vi "Encode Error Listbox.vi"(8 "error in (no error)":errorcluster, 11 "Data":variant) -> (0 "error out":errorcluster, 3 "Encoded Msg":string[](array[string]))   [LabVIEW 2026, in "TALOS.lvlib" / "Guardian.lvlib" / "Guardian.lvclass"]
uses:
  Guardian.lvclass
  Internal uServices/System uServices/Common GUI v3/Common GUI v3/Error Listbox Msg.ctl
  Internal uServices/System uServices/Common GUI v3/Common GUI v3/Error Listbox Msg Action.ctl
  Internal uServices/System uServices/Error Manager/Error Info.ctl
  Internal uServices/System uServices/Common GUI v3/Common GUI v3/Common GUI v3.lvclass
  Internal uServices/System uServices/Error Manager/Error Manager.lvclass
  TALOS.lvlib
  <vilib>/MultiError/TokenizeJSON/Multi Error Cluster.lvlib
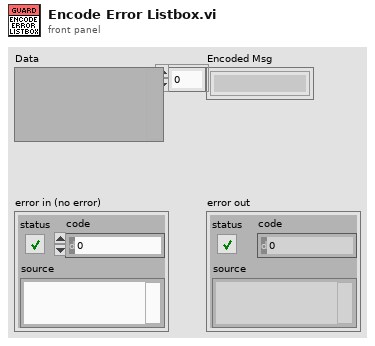
[diagram p1: front panel]
types:
  T1 = typedef "TALOS.lvlib/Common GUI v3.lvlib/Common GUI v3.lvclass/Error Listbox Msg.ctl" = cluster{"Action":T2, "Error Info":T3}
  T2 = typedef "TALOS.lvlib/Common GUI v3.lvlib/Common GUI v3.lvclass/Error Listbox Msg Action.ctl" = enum16{"Add", "Remove", "Clear"}
  T3 = typedef "TALOS.lvlib/Error Manager.lvlib/Error Manager.lvclass/Error Info.ctl" = cluster{"error out":errorcluster, "Time Stamp":timestamp, "Machine Name":string, "GUID":string}
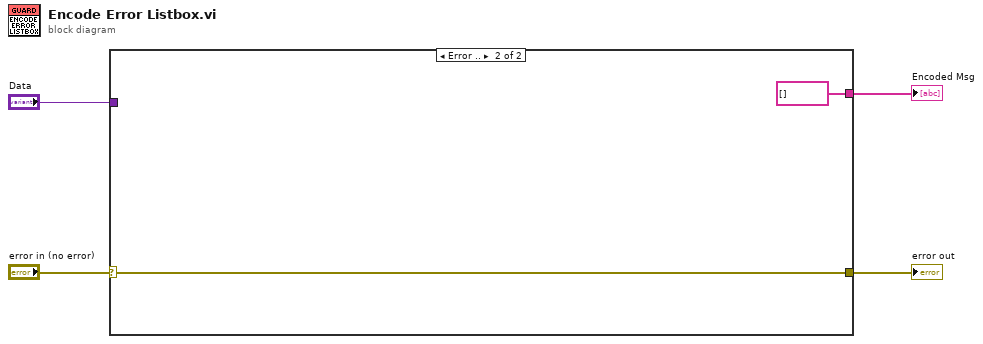
[diagram p0: block diagram]
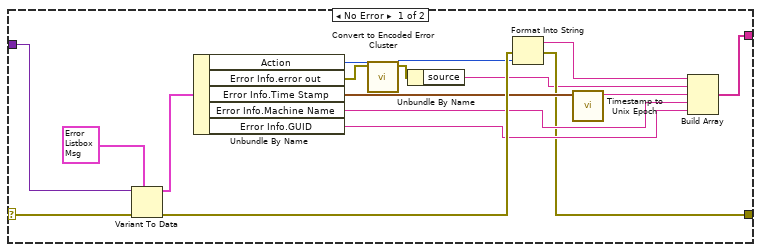
[diagram p2: hidden frame]
diagram:
  n1 = case shown="Error .." "error in (no error)" {
    selector: "error in (no error)" -> [w18 w22]
    tunnel: "Data" -> [w19 _]
    tunnel: [w5 string[] [] ("delimited string")] -> w2
    tunnel: [w9 w22] -> w1
    frame No Error {
      n2 = Variant To Data(error in=w18, type=T1 {"Action"=enum."Add", "Error Info"={"error out"={"status"=FALSE, "code"=0, "source"=""}, "Time Stamp"=timestamp(0 s since 1904-01-01), "Machine Name"="", "GUID"=""}} ("Error Listbox Msg"), Variant=w19) -> (data=w16:T1, error out=w20:errorcluster)
      n3 = Unbundle By Name(w16) -> ("Action"=w15:T2, "Error Info.error out"=w8:errorcluster, "Error Info.Time Stamp"=w14:timestamp, "Error Info.Machine Name"=w11:string, "Error Info.GUID"=w10:string)
      n4 = call <vilib>:"Convert to Encoded Error Cluster.vi"("error in"=w8) -> ("error out"=w7:errorcluster)  [unwired: 10 in]
      n5 = Unbundle By Name(w7) -> ("source"=w6:string)
      n6 = Format Into String(error in=w20, w15) -> (resulting string=w13:string, error out=w9:errorcluster)  [unwired: 2 in]
      n7 = call "Timestamp to Unix Epoch.vi"("seconds since 1Jan1904"=w14) -> ("String"=w12:string)  [unwired: 10 in]
      n8 = Build Array(w13, w6, w12, w11, w10) -> (w5:string[])
    }
    frame Error {
    }
  }
  "Encoded Msg" <- w2
  "error out" <- w1
